vi "Periodic Tasks.vi"(8 "error in":errorcluster) -> ()   [LabVIEW 2016]
doc: "This VI runs in parallel to other tasks. It can contain as many user-defined periodic loops as you need. These can carry out PID or other sorts of timed response."
uses:
  <vilib>/Rock Robotics/WPI/Utilities/WPI_GetSetVariantRefNum.vi
  <vilib>/Rock Robotics/WPI/RobotDrive/WPI_RobotDriveArcadeDrive_Standard(NoSaturation).vi
panel:
  out "Yaw Wind":dbl(graph)
  out "Pitch":dbl(graph)
  out "Roll":dbl(graph)
  out "Yaw":dbl(graph)
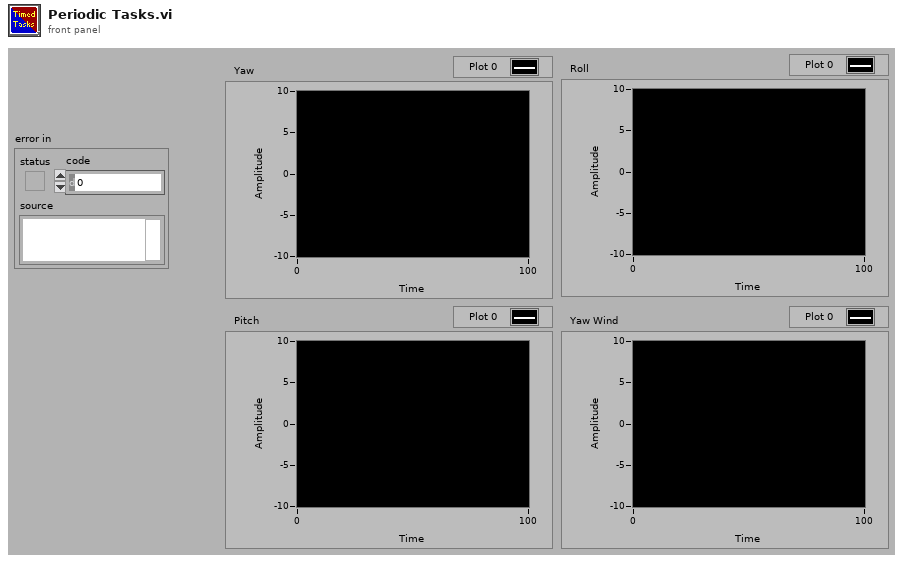
[diagram p1: front panel]
types:
  T1 = typedef "WPI_I2CDevRef.ctl" = cluster{"DevStatus":errorcluster, "Device Address":u8, "Handle":i32, "I2C Bus":T2}
  T2 = typedef "i2c_bus.ctl" = enum16{"I2C On-Board", "I2C MXP", "Invalid"}
  T3 = cluster{"Yaw":dbl, "Roll":dbl, "Pitch":dbl, "Yaw Wind":dbl}
  T4 = typedef "WPI_RobotDriveDevRef.ctl" = cluster{"DevStatus":errorcluster, "Motors[]":T5[], "Square Inputs":bool, "Max Output":dbl}
  T5 = typedef "WPI_MotorControlDeviceRef.ctl" = cluster{"DeviceStatus":errorcluster, "Type":T6, "PWM":cluster{"PWM Channel":T7, "DeadBand":T8}, "CAN":cluster{"Device Number":u8, "SetOutput VI Ref":variant, "GetOutput VI Ref":variant, "Enable VI Ref":variant, "Disable VI Ref":variant, "Data":variant}, "Invert":bool}
  T6 = typedef "WPI_MotorControlType.ctl" = enum16{"PWM", "CAN"}
  T7 = typedef "FPGA_DIOPWMChannel.ctl" = enum8{"PWM 0", "PWM 1", "PWM 2", "PWM 3", "PWM 4", "PWM 5", "PWM 6", "PWM 7", "PWM 8", "PWM 9", "PWM MXP 0", "PWM MXP 1", "PWM MXP 2", "PWM MXP 3", "PWM MXP 4", "PWM MXP 5", "PWM MXP 6", "PWM MXP 7", "PWM MXP 8", "PWM MXP 9", "Invalid"}
  T8 = typedef "WPI_PWMDeadband.ctl" = cluster{"Name":string, "maxPositivePwm":i32, "minPositivePwm":i32, "centerPwm":i32, "maxNegativePwm":i32, "minNegativePwm":i32, "angularRange":u16}
  T9 = typedef "WPI_JoystickDevRef.ctl" = cluster{"Device":T10}
  T10 = typedef "WPI_JoystickDeviceEnum.ctl" = enum16{"USB 0", "USB 1", "USB 2", "USB 3", "USB 4", "USB 5"}
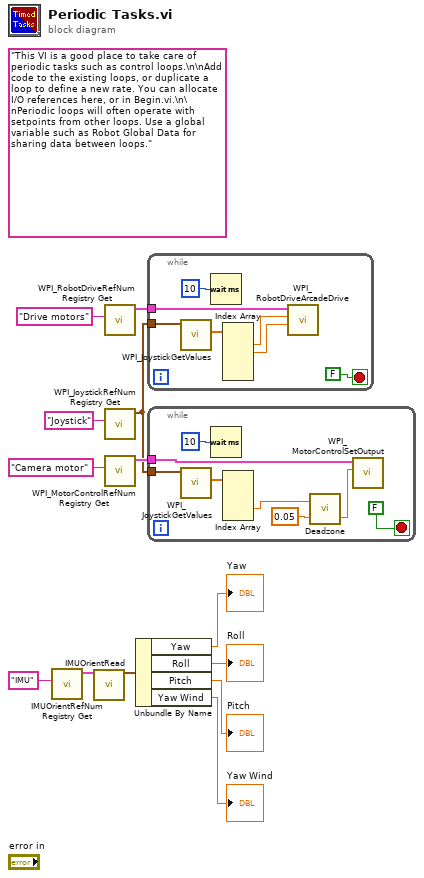
[diagram p0: block diagram]
diagram:
  (unwired) "This VI is a good place to take care of periodic tasks such as control loops.\n\nAdd code to the existing loops, or duplicate a loop to define a new rate. You can allocate I/O references here, or in Begin.vi.\n\nPeriodic loops will often operate with setpoints from other loops. Use a global variable such as Robot Global Data for sharing data between loops."
  n1 = call <userlib>:"IMUOrientRefNum Registry Get.vi"("refnum name"="IMU") -> ("I2CDevRef out"=w6:T1)  [unwired: 9 in, 1 out]
  n2 = call <userlib>:"IMUOrientRead.vi"("I2CDevRef"=w6) -> ("Orient Y/R/P"=w5:T3)  [unwired: 8 in, 6 out]
  n3 = call <vilib>:"WPI_RobotDriveRefNum Registry Get.vi"("refnum name"="Drive motors") -> ("RobotDriveDevRef"=w8:T4)  [unwired: 9 in, 1 out]
  n4 = call <vilib>:"WPI_JoystickRefNum Registry Get.vi"("refnum name"="Joystick") -> ("JoystickDevRef"=w9:T9)  [unwired: 9 in, 1 out]
  n5 = call <vilib>:"WPI_MotorControlRefNum Registry Get.vi"("refnum name"="Camera motor") -> ("MotorControlDevRef"=w10:T5)  [unwired: 9 in, 1 out]
  n6 = Unbundle By Name(w5) -> ("Yaw"=→"Yaw":dbl, "Roll"=→"Roll":dbl, "Pitch"=→"Pitch":dbl, "Yaw Wind"=→"Yaw Wind":dbl)
  n7 = while {
    tunnel: w9 -> [w19]
    tunnel: w8 -> [w20]
    stop <- FALSE stop-if-true
    n8 = call <vilib>:"WPI_JoystickGetValues.vi"("JoystickDevRef"=w19) -> ("Axes"=w18:dbl[])  [unwired: 6 in, 4 out]
    n9 = Wait (ms)(milliseconds to wait=u32 10) -> ()  [unwired: 1 out]
    n10 = Index Array(array=w18) -> (element #1=w16:dbl, element #2=w17:dbl)  [unwired: 5 in, 3 out]
    n11 = call-poly <vilib>:"WPI_RobotDriveArcadeDrive.vi"("Y axis value"=w17, "X axis value"=w16, "RobotDriveDevRef"=w20) -> ()  [unwired: 6 in, 3 out]
  }
  n12 = while {
    tunnel: w10 -> [w28]
    tunnel: w9 -> [w26]
    stop <- FALSE stop-if-true
    n13 = call <vilib>:"WPI_JoystickGetValues.vi"("JoystickDevRef"=w26) -> ("Axes"=w27:dbl[])  [unwired: 6 in, 4 out]
    n14 = Wait (ms)(milliseconds to wait=u32 10) -> ()  [unwired: 1 out]
    n15 = Index Array(array=w27) -> (element #3=w23:dbl)  [unwired: 4 in, 3 out]
    n16 = call <userlib>:"Deadzone.vi"("Deadzone"=0.05, "Input Signal"=w23) -> ("Output Signal"=w21:dbl)  [unwired: 1 out]
    n17 = call <vilib>:"WPI_MotorControlSetOutput.vi"("Output"=w21, "MotorControlDevRef"=w28) -> ()  [unwired: 7 in, 3 out]
  }
